vi "Default controls - load control values.vi"(8 "error in (no error)":errorcluster, 11 "VI's path to save controls":path) -> (0 "error out":errorcluster, 3 "INI's path to the saved controls":path)   [LabVIEW 2020]
uses:
  Save-Load-Defaults.lvlib/Save-Load-Defaults.lvlib
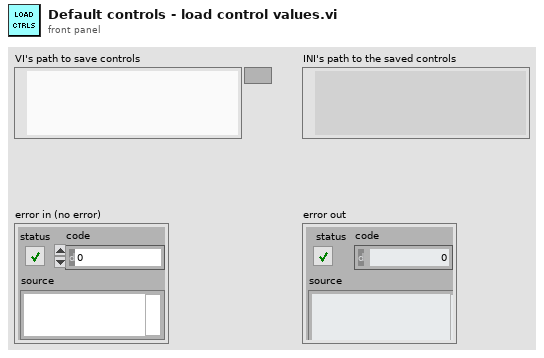
[diagram p1: front panel]
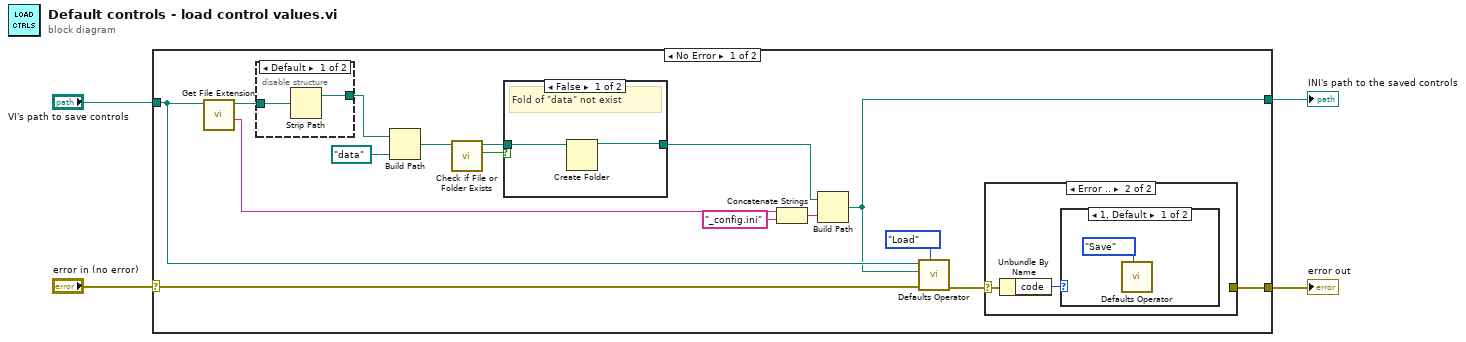
[diagram p0: block diagram]
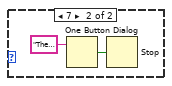
[diagram p4: hidden frame]
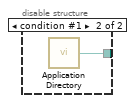
[diagram p5: hidden frame]
diagram:
  n1 = case shown="No Error" "error in (no error)" {
    selector: "error in (no error)" -> [w17 w34]
    tunnel: [w20 w34] -> w4
    tunnel: "VI's path to save controls" -> [w16 w33]
    tunnel: [w12 w33] -> w2
    frame No Error {
      n2 = call <vilib>:"Get File Extension.vi"("file"=w16) -> ("filename without extension"=w14:string, "dup file"=w15:path)  [unwired: 6 in, 3 out]
      n3 = disable-structure shown="Default" {
        disable-tunnel: w15 -> [w31 _]
        disable-tunnel: [w30 w32] -> w10
        frame condition #0 (active) {
          n4 = Strip Path(path=w31) -> (stripped path=w30:path)  [unwired: 1 out]
        }
        frame condition #1 {
          n5 = call <vilib>:"Application Directory.vi"() -> ("Application Directory"=w32:path)
        }
      }
      n6 = Build Path(base path=w10, name or relative path=path "data") -> (appended path=w8:path)
      n7 = call <vilib>:"Check if File or Folder Exists.vi"("path"=w8) -> ("file or folder exists?"=w7:bool, "dup path"=w6:path)  [unwired: 8 in, 1 out]
      n8 = case shown="False" w7 {
        tunnel: w6 -> [w22 w23]
        tunnel: [w21 w23] -> w5
        frame False {
          # "Fold of \"data\" not exist"
          n9 = Create Folder(path (use dialog)=w22) -> (created path=w21:path)  [unwired: 2 in, 2 out]
        }
        frame True {
          # "Folder \"data\" existed"
        }
      }
      n10 = Concatenate Strings(w14, "_config.ini" ("string")) -> (w9:string)
      n11 = Build Path(base path=w5, name or relative path=w9) -> (appended path=w12:path)
      n12 = call "Defaults Operator.vi"("Operation (Load)"=enum16{"Load", "Save"}."Load", "error in (no error)"=w17, "INI's path"=w12, "VI's path"=w16) -> ("error out"=w19:errorcluster)  [unwired: 5 in, 2 out]
      n13 = case shown="Error .." w19 {
        selector: w19 -> [w24 w26]
        tunnel: [w24 _] -> w20
        frame No Error {
        }
        frame Error {
          n14 = Unbundle By Name(w26) -> ("code"=w25:i32)
          n15 = case shown="1, Default" w25 {
            frame 1, Default {
              n16 = call "Defaults Operator.vi"("Operation (Load)"=enum16{"Load", "Save"}."Save") -> ()  [unwired: 8 in, 3 out]
            }
            frame 7 {
              n17 = One Button Dialog(message="The path to INI file or INI format is invalid.\n\nProgram will be quit.\n\n(Error 7)") -> (true=w28:bool)  [unwired: 1 in]
              n18 = Stop(stop? (T)=w28) -> ()
            }
          }
        }
      }
    }
    frame Error {
    }
  }
  "error out" <- w4
  "INI's path to the saved controls" <- w2
